vi "FTW-Tree-ItemToggleOpen.vi"(0 "Tree Ctl Ref":refnum<vi>, 5 "Tag":string, 11 "error in":errorcluster) -> (4 "Tree Ctl Ref out":refnum<vi>, 15 "error out":errorcluster)   [LabVIEW 2012]
panel:
  # "Inputs"
  # "Outputs"
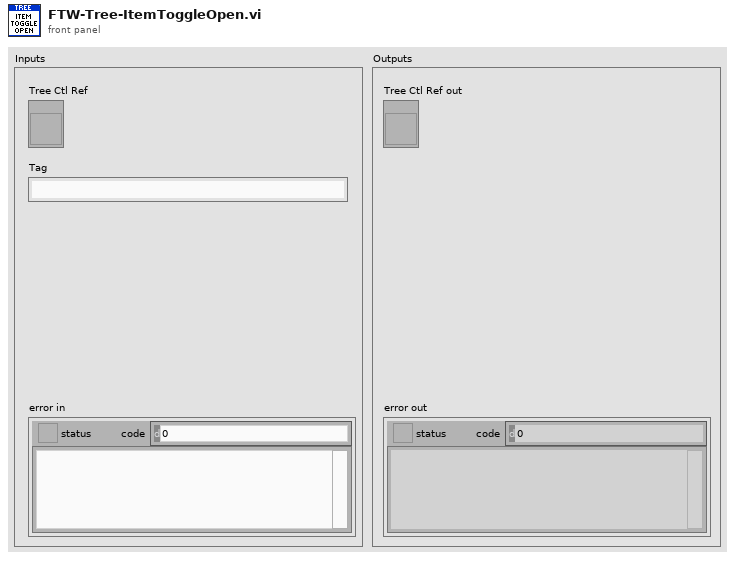
[diagram p1: front panel]
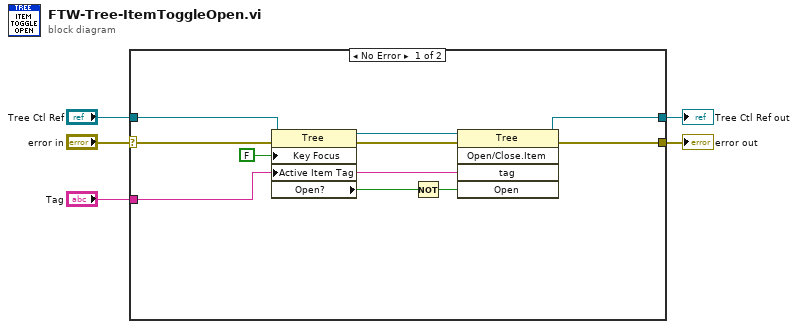
[diagram p0: block diagram]
diagram:
  n1 = case shown="No Error" "error in" {
    selector: "error in" -> [w11 w17]
    tunnel: [w8 w17] -> w5
    tunnel: "Tree Ctl Ref" -> [w12 w16]
    tunnel: "Tag" -> [w7 _]
    tunnel: [w10 w16] -> w2
    frame No Error {
      n2 = property on="Property Node" class="Tree"(reference=w12, error in=w11, "Key Focus"=FALSE, "Active Item Tag"=w7) -> (reference out=w9:refnum<vi>, error out=w15:errorcluster, "Open?"=w14:bool)
      n3 = Not(x=w14) -> (.not. x?=w13:bool)
      n4 = invoke on="Invoke Node" class="Tree" method="Open/Close.Item"(reference=w9, error in=w15, "tag"=w7, "Open"=w13) -> (reference out=w10:refnum<vi>, error out=w8:errorcluster)  [unwired: 1 in, 3 out]
    }
    frame Error {
    }
  }
  "error out" <- w5
  "Tree Ctl Ref out" <- w2
